vi "rs3 delete frame queue2.vi"(8 "error in (no error)":errorcluster, 11 "queue":u64) -> (0 "error out":errorcluster)   [LabVIEW 2017, in "libRealSense3.lvlib"]
doc: "Delete the queue, when done with it."
uses:
  libRealSense3.lvlib
  realsense2.dll
panel:
  # "RS Delete Frame Queue"
  # "(C) Intel Corp. 2017,  AGJ"
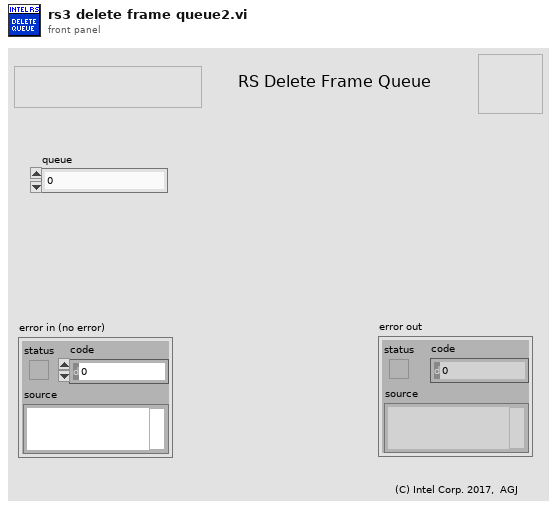
[diagram p1: front panel]
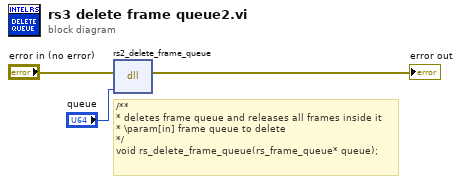
[diagram p0: block diagram]
diagram:
  # "/**\n* deletes frame queue and releases all frames inside it\n* \\param[in] frame queue to delete\n*/\nvoid rs_delete_frame_queue(rs_frame_queue* queue);"
  n1 = dll-call lib="C:/Users/smartek/Desktop/labview/realsense2.dll" fn="rs2_delete_frame_queue"(error in="error in (no error)", "queue"="queue") -> (error out=→"error out":errorcluster)  [unwired: 4 in, 1 out]
